vi "Parse TOML String.vi"(8 "error in (no error)":errorcluster, 11 "String":string) -> (0 "error out":errorcluster, 3 "Table":T1[](array[typedef]))   [LabVIEW 2015, in "TOML.lvlib"]
uses:
  TOML.lvlib
  TOML Key-Value Pair.ctl
  TOML Value.ctl
  Context.ctl
  State.ctl
  Table Context.ctl
  Key-Value Pair.ctl
  Value.ctl
  Table Array Context.ctl
  Array Context.ctl
  <vilib>/regexp/Match Regular Expression.xnode
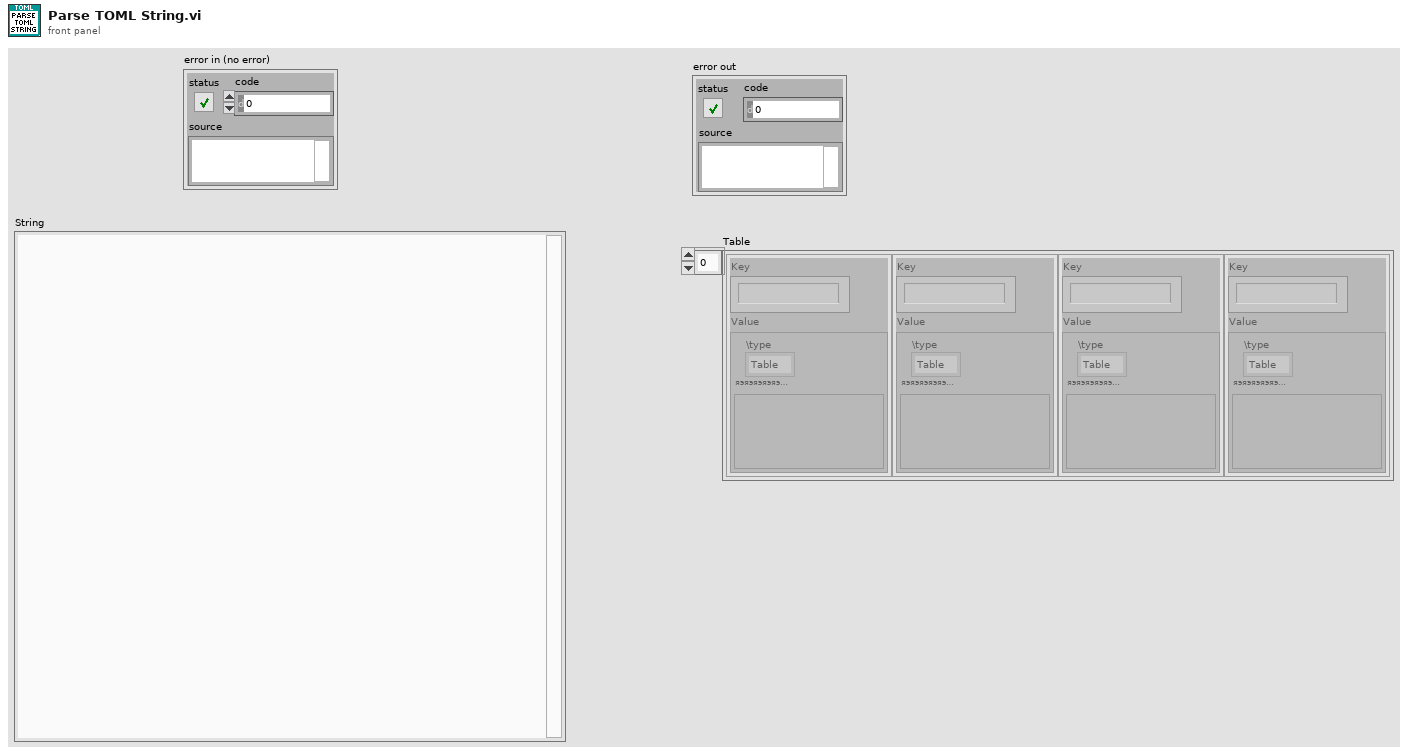
[diagram p1: front panel]
types:
  T1 = typedef "TOML.lvlib/TOML Key-Value Pair.ctl" = cluster{"Key":string, "Value":T2}
  T2 = typedef "TOML.lvlib/TOML Value.ctl" = cluster{"\\type":enum16{"Table", "Array", "String", "Integer", "Float", "Boolean", "Offset Date-Time", "Local Date-Time", "Local Date", "Local Time"}, "яэяэяэяэяэяюяэяэяэ\"TOML.lvlib:TOML Key-Value Pair.ctlяэяэяэяэяэяюяэяэяэTOML.lvlib:TOML Value.ctl$$":variant}
  T3 = typedef "TOML.lvlib/Table Context.ctl" = cluster{"Table":T4[], "Key":string}
  T4 = typedef "TOML.lvlib/Key-Value Pair.ctl" = cluster{"Key":string, "Value":T5}
  T5 = typedef "TOML.lvlib/Value.ctl" = cluster{"Type":enum16{"Table", "Array", "String", "Integer", "Float", "Boolean", "Offset Date-Time", "Local Date-Time", "Local Date", "Local Time"}, "Value":variant}
  T6 = typedef "TOML.lvlib/State.ctl" = enum16{"Table", "Value", "Inline Table"}
  T7 = typedef "TOML.lvlib/Context.ctl" = cluster{"Type":enum16{"Table", "Array", "Inline Table", "Table Array"}, "Value":variant}
  T8 = typedef "TOML.lvlib/Table Array Context.ctl" = cluster{"Table Array":cluster{"Table":T4[]}[], "Index":i32, "Key":string}
  T9 = typedef "TOML.lvlib/Array Context.ctl" = cluster{"Array":T5[], "Index":i32}
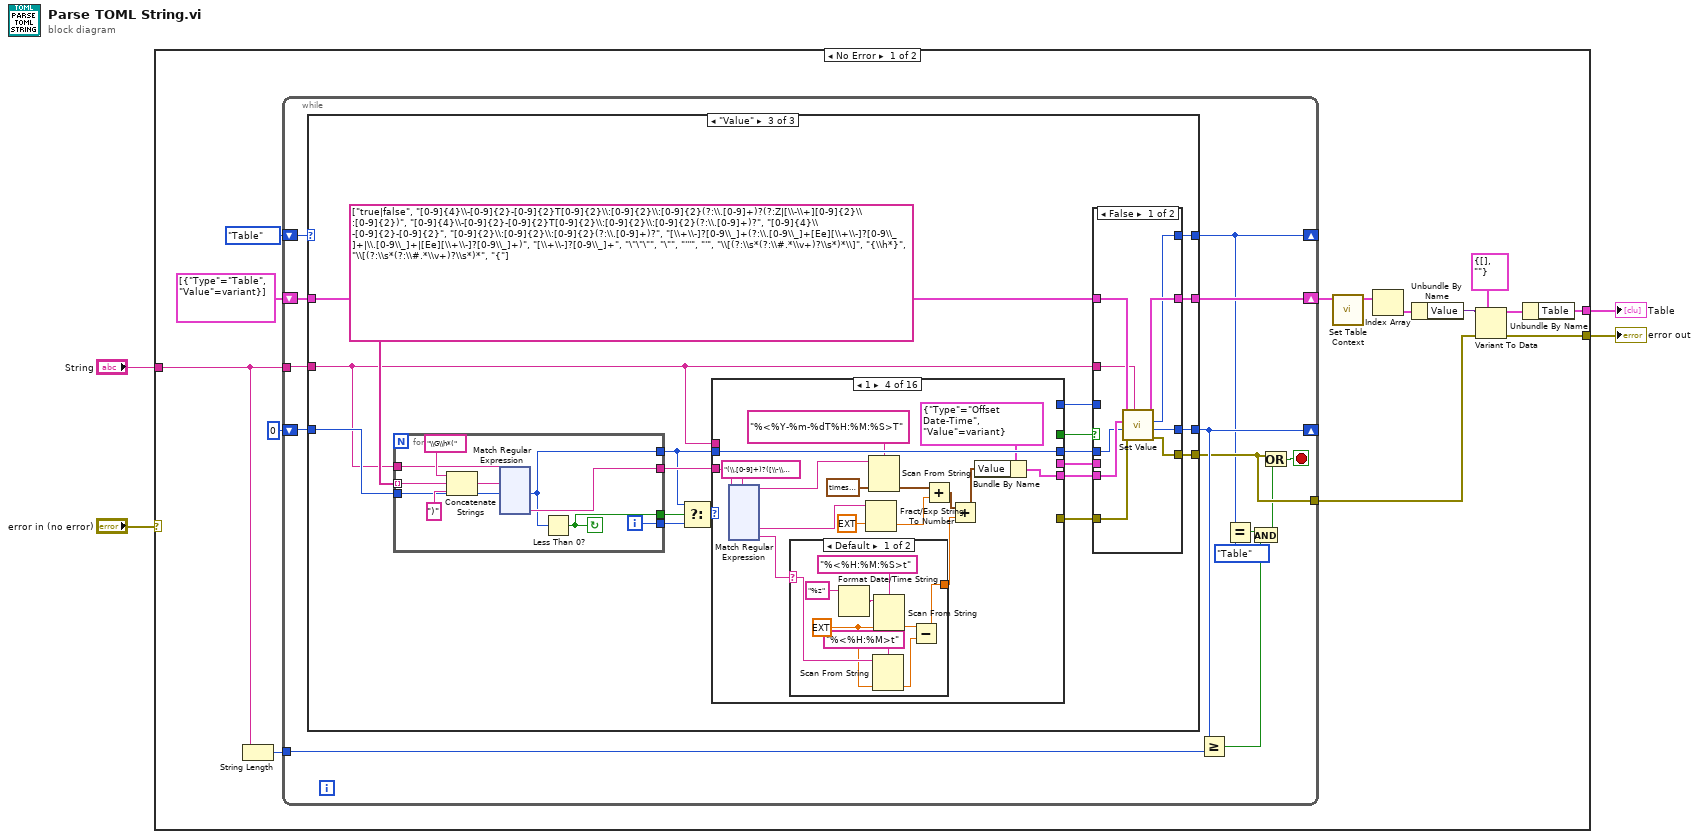
[diagram p0: block diagram]
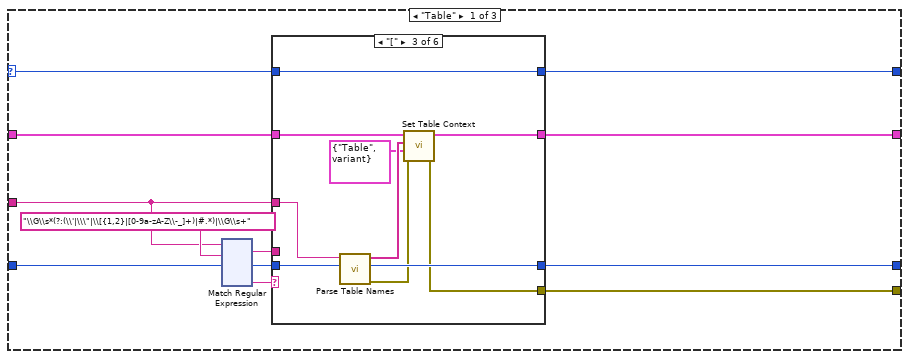
[diagram p2: hidden frame]
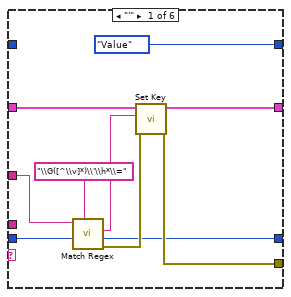
[diagram p3: hidden frame]
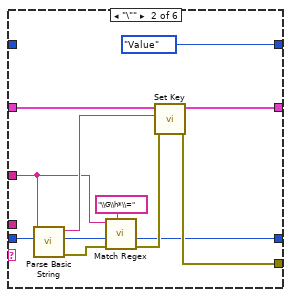
[diagram p4: hidden frame]
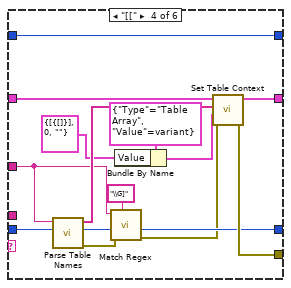
[diagram p5: hidden frame]
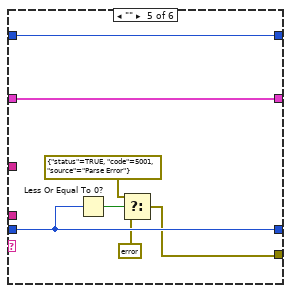
[diagram p6: hidden frame]
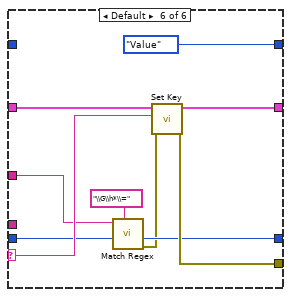
[diagram p7: hidden frame]
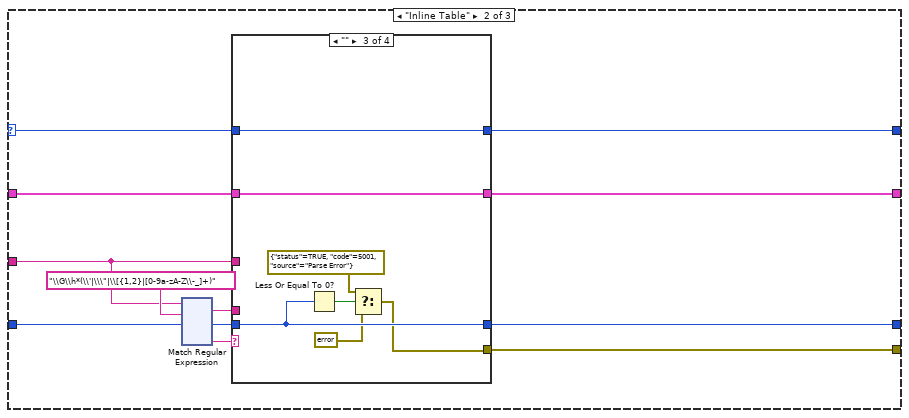
[diagram p8: hidden frame]
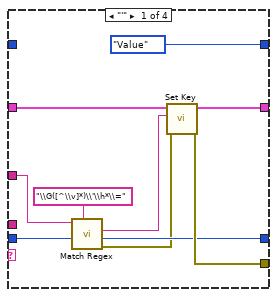
[diagram p9: hidden frame]
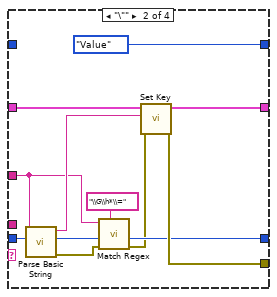
[diagram p10: hidden frame]
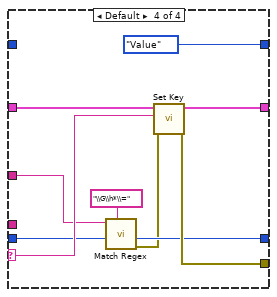
[diagram p11: hidden frame]
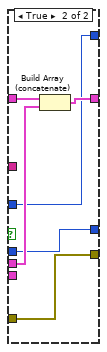
[diagram p12: hidden frame]
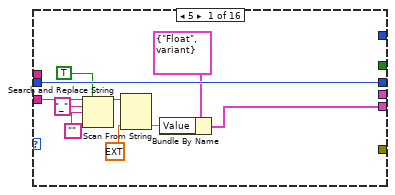
[diagram p13: hidden frame]
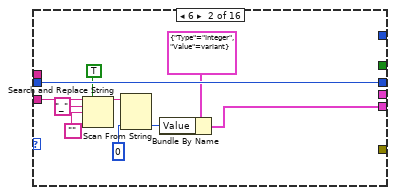
[diagram p14: hidden frame]
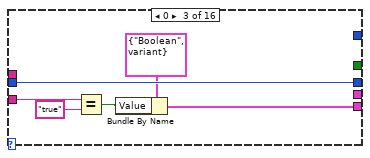
[diagram p15: hidden frame]
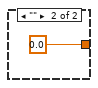
[diagram p16: hidden frame]
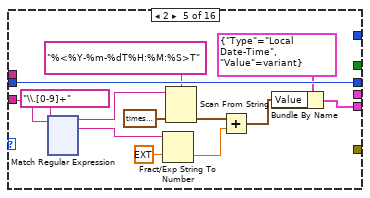
[diagram p17: hidden frame]
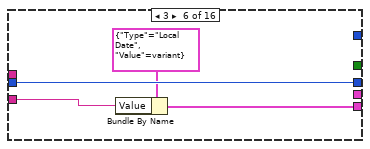
[diagram p18: hidden frame]
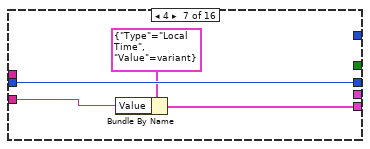
[diagram p19: hidden frame]
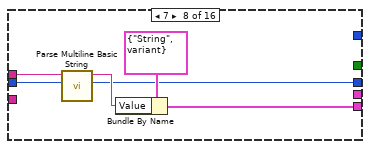
[diagram p20: hidden frame]
diagram:
  n1 = case shown="No Error" "error in (no error)" {
    selector: "error in (no error)" -> [_ w906]
    tunnel: "String" -> [w15 _]
    tunnel: [w7 _] -> w3
    tunnel: [w6 w906] -> w2
    frame No Error {
      n2 = String Length(string=w15) -> (length=w14:i32)
      n3 = while {
        tunnel: w15 -> [w31]
        shift-right: [w21] -> _
        shift-left: State."Table" ("State") -> [w32]
        shift-right: [w29] -> w13
        shift-left: T7[] [{"Type"=enum."Table", "Value"=variant}] -> [w28]
        shift-right: [w24] -> _
        shift-left: 0 -> [w30]
        tunnel: w14 -> [w26]
        tunnel: [w23] -> w5
        stop <- w27 stop-if-true
        n4 = case shown="\"Value\"" w32 {
          selector: w32 -> [w40 w232 _]
          tunnel: w31 -> [w34 w226 w392]
          tunnel: w30 -> [w33 w225 w409]
          tunnel: [w41 w233 w396] -> w21
          tunnel: [w39 w231 w403] -> w29
          tunnel: w28 -> [w38 w230 w402]
          tunnel: [w42 w234 w393] -> w24
          tunnel: [w37 w229 w400] -> w23
          frame "Table" {
            n5 = xnode "Match Regular Expression"("input string"=w34, "regular expression"="\\G\\s*(?:(\\'|\\\"|\\[{1,2}|[0-9a-zA-Z\\-_]+)|#.*)|\\G\\s+", "offset (0)"=w33) -> ("whole match"=w35:string, "offset past match"=w43:i32, "submatch 1"=w36:string)  [unwired: 3 in, 3 out]
            n6 = case shown="\"[\"" w36 {
              selector: w36 -> [_ _ _ _ _ w104]
              tunnel: [w45 w55 w73 w82 w96 w100] -> w42
              tunnel: w43 -> [w46 w66 w74 w90 w96 w101]
              tunnel: [State."Value" ("State") State."Value" ("State") w76 w91 w98 State."Value" ("State")] -> w41
              tunnel: w40 -> [_ _ w76 w91 w98 _]
              tunnel: [w50 w62 w71 w88 w97 w105] -> w39
              tunnel: w38 -> [w53 w63 w72 w89 w97 w106]
              tunnel: [w51 w64 w67 w86 w92 w107] -> w37
              tunnel: w34 -> [w47 w59 w75 w84 _ w102]
              tunnel: w35 -> [_ _ _ _ _ _]
              frame "'" {
                n7 = call "Match Regex.vi"("regular expression"="\\G([^\\v]*)\\'\\h*\\=", "offset"=w46, "String"=w47) -> ("error out"=w52:errorcluster, "offset past match"=w45:i32, "submatch 1"=w48:string)  [unwired: 5 in, 1 out]
                n8 = call "Set Key.vi"("error in (no error)"=w52, "Key"=w48, "Stack in"=w53) -> ("error out"=w51:errorcluster, "Stack out"=w50:T7[])  [unwired: 7 in]
              }
              frame "\"" {
                n9 = call "Parse Basic String.vi"("start at"=w66, "TOML String"=w59) -> ("error out"=w57:errorcluster, "offset past match"=w58:i32, "String"=w61:string)  [unwired: 7 in]
                n10 = call "Match Regex.vi"("regular expression"="\\G\\h*\\=", "error in (no error)"=w57, "offset"=w58, "String"=w59) -> ("error out"=w56:errorcluster, "offset past match"=w55:i32)  [unwired: 4 in, 2 out]
                n11 = call "Set Key.vi"("error in (no error)"=w56, "Key"=w61, "Stack in"=w63) -> ("error out"=w64:errorcluster, "Stack out"=w62:T7[])  [unwired: 7 in]
              }
              frame "[" {
                n12 = call "Parse Table Names.vi"("start at"=w74, "TOML String"=w75) -> ("error out"=w68:errorcluster, "offset past match"=w73:i32, "Table Stack"=w70:string[])  [unwired: 7 in]
                n13 = call "Set Table Context.vi"("error in (no error)"=w68, "Context"=T7 {"Type"=enum."Table", "Value"=variant}, "Table Names"=w70, "Stack in"=w72) -> ("error out"=w67:errorcluster, "Stack out"=w71:T7[])  [unwired: 6 in]
              }
              frame "[[" {
                n14 = call "Parse Table Names.vi"("start at"=w90, "TOML String"=w84) -> ("error out"=w81:errorcluster, "offset past match"=w83:i32, "Table Stack"=w87:string[])  [unwired: 7 in]
                n15 = call "Match Regex.vi"("regular expression"="\\G]", "error in (no error)"=w81, "offset"=w83, "String"=w84) -> ("error out"=w80:errorcluster, "offset past match"=w82:i32)  [unwired: 4 in, 2 out]
                n16 = Bundle By Name(cluster=T7 {"Type"=enum."Table Array", "Value"=variant} ("Context"), "Value"=T8 {"Table Array"=[{"Table"=[]}], "Index"=0, "Key"=""} ("Table Array Context")) -> (w78:T7)
                n17 = call "Set Table Context.vi"("error in (no error)"=w80, "Context"=w78, "Table Names"=w87, "Stack in"=w89) -> ("error out"=w86:errorcluster, "Stack out"=w88:T7[])  [unwired: 6 in]
              }
              frame "" {
                n18 = Less Or Equal To 0?(x=w96) -> (x <= 0?=w95:bool)
                n19 = Select(t=errorcluster {"status"=TRUE, "code"=5001, "source"="Parse Error"} ("error constant"), s=w95, f=errorcluster {"status"=FALSE, "code"=0, "source"=""}) -> (s? t:f=w92:errorcluster)
              }
              frame Default {
                n20 = call "Match Regex.vi"("regular expression"="\\G\\h*\\=", "offset"=w101, "String"=w102) -> ("error out"=w99:errorcluster, "offset past match"=w100:i32)  [unwired: 5 in, 2 out]
                n21 = call "Set Key.vi"("error in (no error)"=w99, "Key"=w104, "Stack in"=w106) -> ("error out"=w107:errorcluster, "Stack out"=w105:T7[])  [unwired: 7 in]
              }
            }
          }
          frame "Inline Table" {
            n22 = xnode "Match Regular Expression"("input string"=w226, "regular expression"="\\G\\h*(\\'|\\\"|\\[{1,2}|[0-9a-zA-Z\\-_]+)", "offset (0)"=w225) -> ("whole match"=w227:string, "offset past match"=w235:i32, "submatch 1"=w228:string)  [unwired: 3 in, 3 out]
            n23 = case shown="\"\"" w228 {
              selector: w228 -> [_ _ _ w271]
              tunnel: [w239 w251 w264 w267] -> w234
              tunnel: w235 -> [w240 w258 w264 w268]
              tunnel: [State."Value" ("State") State."Value" ("State") w259 State."Value" ("State")] -> w233
              tunnel: w232 -> [_ _ w259 _]
              tunnel: [w243 w254 w265 w272] -> w231
              tunnel: w230 -> [w245 w255 w265 w273]
              tunnel: [w244 w256 w260 w274] -> w229
              tunnel: w226 -> [w241 w250 _ w269]
              tunnel: w227 -> [_ _ _ _]
              frame "'" {
                n24 = call "Match Regex.vi"("regular expression"="\\G([^\\v]*)\\'\\h*\\=", "offset"=w240, "String"=w241) -> ("error out"=w237:errorcluster, "offset past match"=w239:i32, "submatch 1"=w238:string)  [unwired: 5 in, 1 out]
                n25 = call "Set Key.vi"("error in (no error)"=w237, "Key"=w238, "Stack in"=w245) -> ("error out"=w244:errorcluster, "Stack out"=w243:T7[])  [unwired: 7 in]
              }
              frame "\"" {
                n26 = call "Parse Basic String.vi"("start at"=w258, "TOML String"=w250) -> ("error out"=w247:errorcluster, "offset past match"=w252:i32, "String"=w253:string)  [unwired: 7 in]
                n27 = call "Match Regex.vi"("regular expression"="\\G\\h*\\=", "error in (no error)"=w247, "offset"=w252, "String"=w250) -> ("error out"=w248:errorcluster, "offset past match"=w251:i32)  [unwired: 4 in, 2 out]
                n28 = call "Set Key.vi"("error in (no error)"=w248, "Key"=w253, "Stack in"=w255) -> ("error out"=w256:errorcluster, "Stack out"=w254:T7[])  [unwired: 7 in]
              }
              frame "" {
                n29 = Less Or Equal To 0?(x=w264) -> (x <= 0?=w263:bool)
                n30 = Select(t=errorcluster {"status"=TRUE, "code"=5001, "source"="Parse Error"} ("error constant"), s=w263, f=errorcluster {"status"=FALSE, "code"=0, "source"=""}) -> (s? t:f=w260:errorcluster)
              }
              frame Default {
                n31 = call "Match Regex.vi"("regular expression"="\\G\\h*\\=", "offset"=w268, "String"=w269) -> ("error out"=w266:errorcluster, "offset past match"=w267:i32)  [unwired: 5 in, 2 out]
                n32 = call "Set Key.vi"("error in (no error)"=w266, "Key"=w271, "Stack in"=w273) -> ("error out"=w274:errorcluster, "Stack out"=w272:T7[])  [unwired: 7 in]
              }
            }
          }
          frame "Value" {
            n33 = for {
              tunnel: string[] ["true|false", "[0-9]{4}\\-[0-9]{2}-[0-9]{2}T[0-9]{2}\\:[0-9]{2}\\:[0-9]{2}(?:\\.[0-9]+)?(?:Z|[\\-\\+][0-9]{2}\\:[0-9]{2})", "[0-9]{4}\\-[0-9]{2}-[0-9]{2}T[0-9]{2}\\:[0-9]{2}\\:[0-9]{2}(?:\\.[0-9]+)?", "[0-9]{4}\\-[0-9]{2}-[0-9]{2}", "[0-9]{2}\\:[0-9]{2}\\:[0-9]{2}(?:\\.[0-9]+)?", "[\\+\\-]?[0-9\\_]+(?:\\.[0-9\\_]+[Ee][\\+\\-]?[0-9\\_]+|\\.[0-9\\_]+|[Ee][\\+\\-]?[0-9\\_]+)", "[\\+\\-]?[0-9\\_]+", "\"\"\"", "\"", "'''", "'", "\\[(?:\\s*(?:\\#.*\\v+)?\\s*)*\\]", "{\\h*}", "\\[(?:\\s*(?:\\#.*\\v+)?\\s*)*", "{"] -> [w789] mode=indexing
              tunnel: w392 -> [w785]
              tunnel: w409 -> [w784]
              tunnel: [w783] -> w405
              tunnel: [w782] -> w404
              tunnel: [w781] -> w408
              tunnel: [w780] -> w407
              i -> [w780]
              stop <- w781 continue-if-true
              n34 = Concatenate Strings("\\G\\h*(" ("string"), w789, ")" ("string")) -> (w786:string)
              n35 = xnode "Match Regular Expression"("input string"=w785, "regular expression"=w786, "offset (0)"=w784) -> ("offset past match"=w782:i32, "submatch 1"=w783:string)  [unwired: 3 in, 4 out]
              n36 = Less Than 0?(x=w782) -> (x < 0?=w781:bool)
            }
            n37 = Select(t=w404, s=w408, f=w407) -> (s? t:f=w406:i32)
            n38 = case shown="1" w406 {
              tunnel: w405 -> [w430 w440 w450 w452 w597 w722 w726 _ _ _ _ _ _ _ _ _]
              tunnel: w404 -> [w435 w445 w451 w467 w607 w725 w729 w731 w738 w746 w751 w755 w762 w771 w777 w779]
              tunnel: [w435 w445 w451 w467 w607 w725 w729 w730 w737 w747 w751 w755 w759 w771 w777 w779] -> w394
              tunnel: [_ _ _ _ _ _ _ _ _ w744 _ _ w758 _ _ errorcluster {"status"=TRUE, "code"=5001, "source"=""} ("error constant")] -> w401
              tunnel: [w431 w441 w446 w465 w605 w723 w727 w734 w740 w748 w752 w756 w764 _ _ _] -> w399
              tunnel: w392 -> [_ _ _ _ _ _ _ w733 w739 w743 _ _ w761 _ _ _]
              tunnel: [_ _ _ _ _ _ _ _ _ _ _ _ _ TRUE TRUE _] -> w398
              tunnel: [_ _ _ _ _ _ _ _ _ _ _ _ _ w767 w774 _] -> w397
              tunnel: [_ _ _ _ _ _ _ _ _ _ _ _ _ State."Value" ("State") State."Inline Table" ("State") _] -> w395
              frame 5 {
                n39 = Search and Replace String(replace all?=TRUE ("replace all? (F)"), input string=w430, search string="_", replace string="") -> (result string=w429:string)  [unwired: 4 in, 3 out]
                n40 = Scan From String(input string=w429, default 1=ext 0.0 ("default value 1")) -> (output 1=w433:ext)  [unwired: 3 in, 3 out]
                n41 = Bundle By Name(cluster=T5 {"Type"=enum."Float", "Value"=variant} ("Value"), "Value"=w433) -> (w431:T5)
              }
              frame 6 {
                n42 = Search and Replace String(replace all?=TRUE ("replace all? (F)"), input string=w440, search string="_", replace string="") -> (result string=w439:string)  [unwired: 4 in, 3 out]
                n43 = Scan From String(input string=w439, default 1=i64 0 ("default value 1")) -> (output 1=w443:i64)  [unwired: 3 in, 3 out]
                n44 = Bundle By Name(cluster=T5 {"Type"=enum."Integer", "Value"=variant} ("Value"), "Value"=w443) -> (w441:T5)
              }
              frame 0 {
                n45 = Equal?(x=w450, y="true") -> (x = y?=w447:bool)
                n46 = Bundle By Name(cluster=T5 {"Type"=enum."Boolean", "Value"=variant} ("Value"), "Value"=w447) -> (w446:T5)
              }
              frame 1 {
                n47 = xnode "Match Regular Expression"("input string"=w452, "regular expression"="(\\.[0-9]+)?([\\-\\+][0-9]{2}\\:[0-9]{2})?Z?$") -> ("before match"=w458:string, "submatch 1"=w457:string, "submatch 2"=w454:string)  [unwired: 4 in, 4 out]
                n48 = case shown="Default" w454 {
                  selector: w454 -> [w473 _]
                  tunnel: [w470 0.0] -> w453
                  frame Default {
                    w468 = ext 0.0 ("default value 1")
                    n49 = Format Date/Time String(time format string (%c)="%z") -> (date/time string=w475:string)  [unwired: 2 in]
                    n50 = Scan From String(format string="%<%H:%M>t", input string=w473, default 1=w468) -> (output 1=w471:ext)  [unwired: 2 in, 3 out]
                    n51 = Scan From String(format string="%<%H:%M:%S>t", input string=w475, default 1=w468) -> (output 1=w472:ext)  [unwired: 2 in, 3 out]
                    n52 = Subtract(x=w472, y=w471) -> (x-y=w470:ext)
                  }
                  frame "" {
                  }
                }
                n53 = Fract/Exp String To Number(string=w457, default (0 dbl)=ext 0.0 ("default (0 DBL)")) -> (number=w459:ext)  [unwired: 2 in, 1 out]
                n54 = Scan From String(format string="%<%Y-%m-%dT%H:%M:%S>T", input string=w458, default 1=timestamp(0 s since 1904-01-01)) -> (output 1=w460:timestamp)  [unwired: 2 in, 3 out]
                n55 = Add(x=w460, y=w459) -> (x+y=w456:timestamp)
                n56 = Add(x=w456, y=w453) -> (x+y=w455:timestamp)
                n57 = Bundle By Name(cluster=T5 {"Type"=enum."Offset Date-Time", "Value"=variant} ("Value"), "Value"=w455) -> (w465:T5)
              }
              frame 2 {
                n58 = xnode "Match Regular Expression"("input string"=w597, "regular expression"="\\.[0-9]+") -> ("before match"=w598:string, "whole match"=w595:string)  [unwired: 4 in, 3 out]
                n59 = Fract/Exp String To Number(string=w595, default (0 dbl)=ext 0.0 ("default (0 DBL)")) -> (number=w599:ext)  [unwired: 2 in, 1 out]
                n60 = Scan From String(format string="%<%Y-%m-%dT%H:%M:%S>T", input string=w598, default 1=timestamp(0 s since 1904-01-01)) -> (output 1=w600:timestamp)  [unwired: 2 in, 3 out]
                n61 = Add(x=w600, y=w599) -> (x+y=w596:timestamp)
                n62 = Bundle By Name(cluster=T5 {"Type"=enum."Local Date-Time", "Value"=variant} ("Value"), "Value"=w596) -> (w605:T5)
              }
              frame 3 {
                n63 = Bundle By Name(cluster=T5 {"Type"=enum."Local Date", "Value"=variant} ("Value"), "Value"=w722) -> (w723:T5)
              }
              frame 4 {
                n64 = Bundle By Name(cluster=T5 {"Type"=enum."Local Time", "Value"=variant} ("Value"), "Value"=w726) -> (w727:T5)
              }
              frame 7 {
                n65 = call "Parse Multiline Basic String.vi"("start at"=w731, "TOML String"=w733) -> ("offset past match"=w730:i32, "String"=w732:string)  [unwired: 7 in, 1 out]
                n66 = Bundle By Name(cluster=T5 {"Type"=enum."String", "Value"=variant} ("Value"), "Value"=w732) -> (w734:T5)
              }
              frame 8 {
                n67 = call "Parse Basic String.vi"("start at"=w738, "TOML String"=w739) -> ("offset past match"=w737:i32, "String"=w736:string)  [unwired: 7 in, 1 out]
                n68 = Bundle By Name(cluster=T5 {"Type"=enum."String", "Value"=variant} ("Value"), "Value"=w736) -> (w740:T5)
              }
              frame 10 {
                n69 = call "Match Regex.vi"("regular expression"="\\G([^\\v]*)\\'", "offset"=w746, "String"=w743) -> ("error out"=w744:errorcluster, "offset past match"=w747:i32, "submatch 1"=w745:string)  [unwired: 5 in, 1 out]
                n70 = Bundle By Name(cluster=T5 {"Type"=enum."String", "Value"=variant} ("Value"), "Value"=w745) -> (w748:T5)
              }
              frame 11 {
                n71 = Bundle By Name(cluster=T5 {"Type"=enum."Array", "Value"=variant} ("Value"), "Value"=T5[] []) -> (w752:T5)
              }
              frame 12 {
                n72 = Bundle By Name(cluster=T5 {"Type"=enum."Table", "Value"=variant} ("Value"), "Value"=T4[] []) -> (w756:T5)
              }
              frame 9 {
                n73 = call "Match Regex.vi"("regular expression"="\\G\\r?\\n?((?s:.)*?)'''", "offset"=w762, "String"=w761) -> ("error out"=w758:errorcluster, "offset past match"=w759:i32, "submatch 1"=w763:string)  [unwired: 5 in, 1 out]
                n74 = Bundle By Name(cluster=T5 {"Type"=enum."String", "Value"=variant} ("Value"), "Value"=w763) -> (w764:T5)
              }
              frame 13 {
                n75 = Bundle By Name(cluster=T7 {"Type"=enum."Array", "Value"=variant} ("Context"), "Value"=T9 {"Array"=[], "Index"=0} ("Array Context")) -> (w767:T7)
              }
              frame 14 {
                n76 = Bundle By Name(cluster=T7 {"Type"=enum."Inline Table", "Value"=variant} ("Context"), "Value"=T3 {"Table"=[], "Key"=""} ("Table Context")) -> (w774:T7)
              }
              frame Default {
              }
            }
            n77 = case shown="False" w398 {
              tunnel: [w419 w423] -> w403
              tunnel: w402 -> [w418 w424]
              tunnel: w401 -> [w417 w425]
              tunnel: [w416 w425] -> w400
              tunnel: w399 -> [w415 _]
              tunnel: w397 -> [_ w422]
              tunnel: [w414 w421] -> w396
              tunnel: w395 -> [_ w421]
              tunnel: w394 -> [w413 w420]
              tunnel: [w412 w420] -> w393
              tunnel: w392 -> [w411 _]
              frame False {
                n78 = call "Set Value.vi"("TOML string"=w411, "error in (no error)"=w417, "start position"=w413, "Value"=w415, "Context in"=w418) -> ("error out"=w416:errorcluster, "offset past match"=w412:i32, "State"=w414:T6, "Context out"=w419:T7[])  [unwired: 3 in]
              }
              frame True {
                n79 = Build Array (concatenate)(w424, w422) -> (w423:T7[])
              }
            }
          }
        }
        n80 = Greater Or Equal?(x=w24, y=w26) -> (x >= y?=w25:bool)
        n81 = Equal?(x=w21, y=State."Table") -> (x = y?=w19:bool)
        n82 = And(x=w19, y=w25) -> (x .and. y?=w22:bool)
        n83 = Or(x=w23, y=w22) -> (x .or. y?=w27:bool)
      }
      n84 = call "Set Table Context.vi"("Stack in"=w13) -> ("Stack out"=w12:T7[])  [unwired: 9 in, 1 out]
      n85 = Index Array(array=w12) -> (element=w10:T7)  [unwired: 1 in]
      n86 = Unbundle By Name(w10) -> ("Value"=w9:variant)
      n87 = Variant To Data(error in=w5, type=T3 {"Table"=[], "Key"=""} ("Table Context"), Variant=w9) -> (data=w8:T3, error out=w6:errorcluster)
      n88 = Unbundle By Name(w8) -> ("Table"=w7:T4[])
    }
    frame Error {
    }
  }
  "error out" <- w2
  "Table" <- w3
